vi "FormCalibra7.vi"() -> ()   [LabVIEW 2014]
uses:
  testMachine.ctl
  mainMachine.ctl
  <vilib>/Instr/_visa.llb/VISA Configure Serial Port (Instr).vi
  <vilib>/express/express shared/transition.llb/Dynamic To Waveform Array.vi
  <vilib>/express/express signal manip/GetorSetDDTAttributes/Set DDT Attributes/SetT0.vi
  <vilib>/express/express shared/transition.llb/Waveform Array To Dynamic.vi
  <vilib>/express/express signal manip/GetorSetDDTAttributes/Set DDT Attributes/Set DDT Properties.xnode
panel:
  out "String":string
  in  "VISA Serial Port":refnum<visa-resource-name>
  out "editDistance":dbl caption="Distancia (m)" format="%#_4f"
  in  "Lower level":dbl
  in  "hysteresis":dbl format="%.2p"
  in  "level":dbl format="%.2p"
  out "editTotalWaitLimit":u8
  out "editCountWaitLimit":u8
  out "ledWaitState":bool caption="Wait State"
  out "sliderWaitUpperTime":u8(slide) max=50 scale=0.0..30.0
  out "slideWaitLowerTime":u8(slide) max=30 scale=0.0..1.0
  out "slideWaitTime":u8(slide) scale=0.0..1.0
  out "labelTestTime":string caption="Tempo total de ensaio"
  in  "buttonAcquisition":bool
  in  "editSetWaitTime":u8 caption="Tempo entre ciclos (s)" step=1 format="%0d"
  in  "stop":bool
  out "ledAcquireState":bool caption="Acquire State"
  out "editTotalLowerLimit":u8
  out "editCountLowerLimit":u8
  out "editTotalUpperLimit":u8
  out "editCountUpperLimit":u8
  out "ledEnsaio 3":bool
  out "ledBrakeState":bool caption="Brake State"
  out "ledExitState":bool caption="Exit State"
  out "ledMotorState":bool caption="Motor State"
  out "ledInit2State":bool caption="Init State"
  out "ledBlockState":bool caption="Block State"
  out "ledRunningState":bool caption="Running State"
  out "ledReadyState":bool caption="Ready State"
  out "ledInitState":bool caption="Init State"
  out "mainMachine":T1
  out "testMachine":T2=enum."finish"
  in  "editSetPathToFile":path
  in  "buttonStop":bool
  in  "buttonStart":bool
  out "graphForce":dynamicdata(graph)
  in  "editOffsetForce":dbl caption="Tara" min=0.0 max=100.0 step=0.1
  in  "editSetForce":dbl caption="Fator de conversão"
  out "editForce":dbl caption="Força (Kgf)" format="%#_4f"
  out "graphSpeed":dynamicdata(graph)
  in  "editSetSpeed":dbl caption="Fator de conversão"
  out "editSpeed":dbl caption="Velocidade (km/h)" format="%#_4f"
  out "editEngineSpeed":dbl caption="Rotação (RPM)" format="%#_4f"
  in  "buttonMotor":bool
  in  "buttonBrake":bool
  in  "editSetWaitLowerTime":u8 caption="Tempo de espera (s)"
  in  "editSetWaitUpperTime":u8=3 caption="Tempo de espera (s)"
  in  "editSetNumberOfCycles":u16 caption="Número de ciclos" max=999 step=1 format="%0d"
  in  "editSetLowerLimit":u32 caption="Limite inferior (km/h)"
  in  "editSetUpperLimit":u32 caption="Limite superior (km/h)"
  out "editTempA":dbl caption="Temperatura A (ºC)"
  in  "editSetTempRef":dbl caption="Offset referência" step=0.01 format="%#_2f"
  out "editTempRef":dbl caption="Referência (ºC)"
  out "ledMotor":bool
  out "ledBrake":bool
  out "ledEnsaio":bool
  out "labelTotalCycle":string
  out "labelCurrentCycle":string
  out "labelSystemTitle":string
  in  "editCurrCycleCtr":u32
  in  "velocidade 2":u32
  out "velocidade":u32
  # "Bancada de Frenagem - Ensaio"
  # "Ensaio"
  # "Temperatura"
  # "Rotação"
  # "Célula de Carga"
  # "Configurações do ensaio"
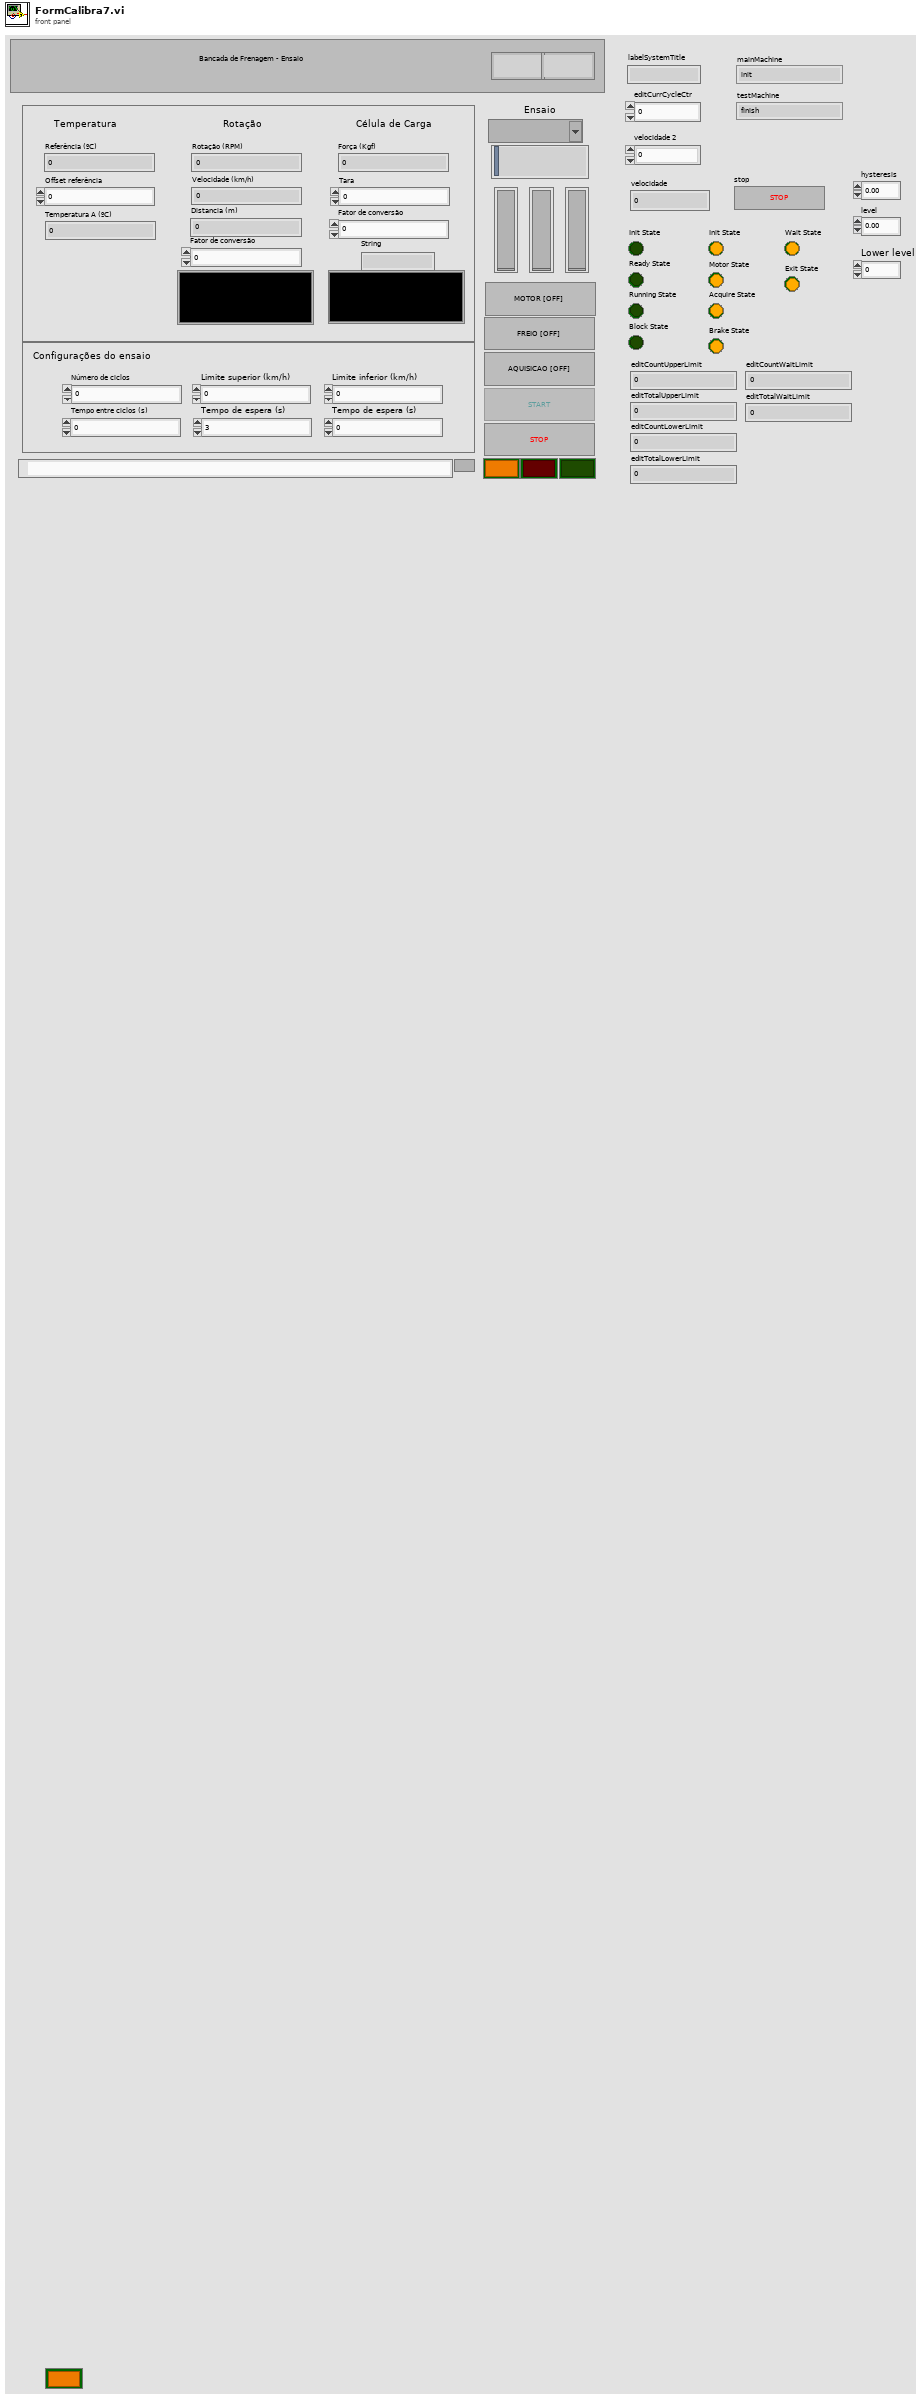
[diagram p1: front panel]
types:
  T1 = typedef "mainMachine.ctl" = enum16{"init", "ready", "running", "blocked", "finish"}
  T2 = typedef "testMachine.ctl" = enum16{"init", "motor", "motor acquire", "brake", "brake acquire", "wait ", "finish", "exit"}
  T3 = enum8{"Enabled", "Disabled", "Disabled and Grayed Out"}
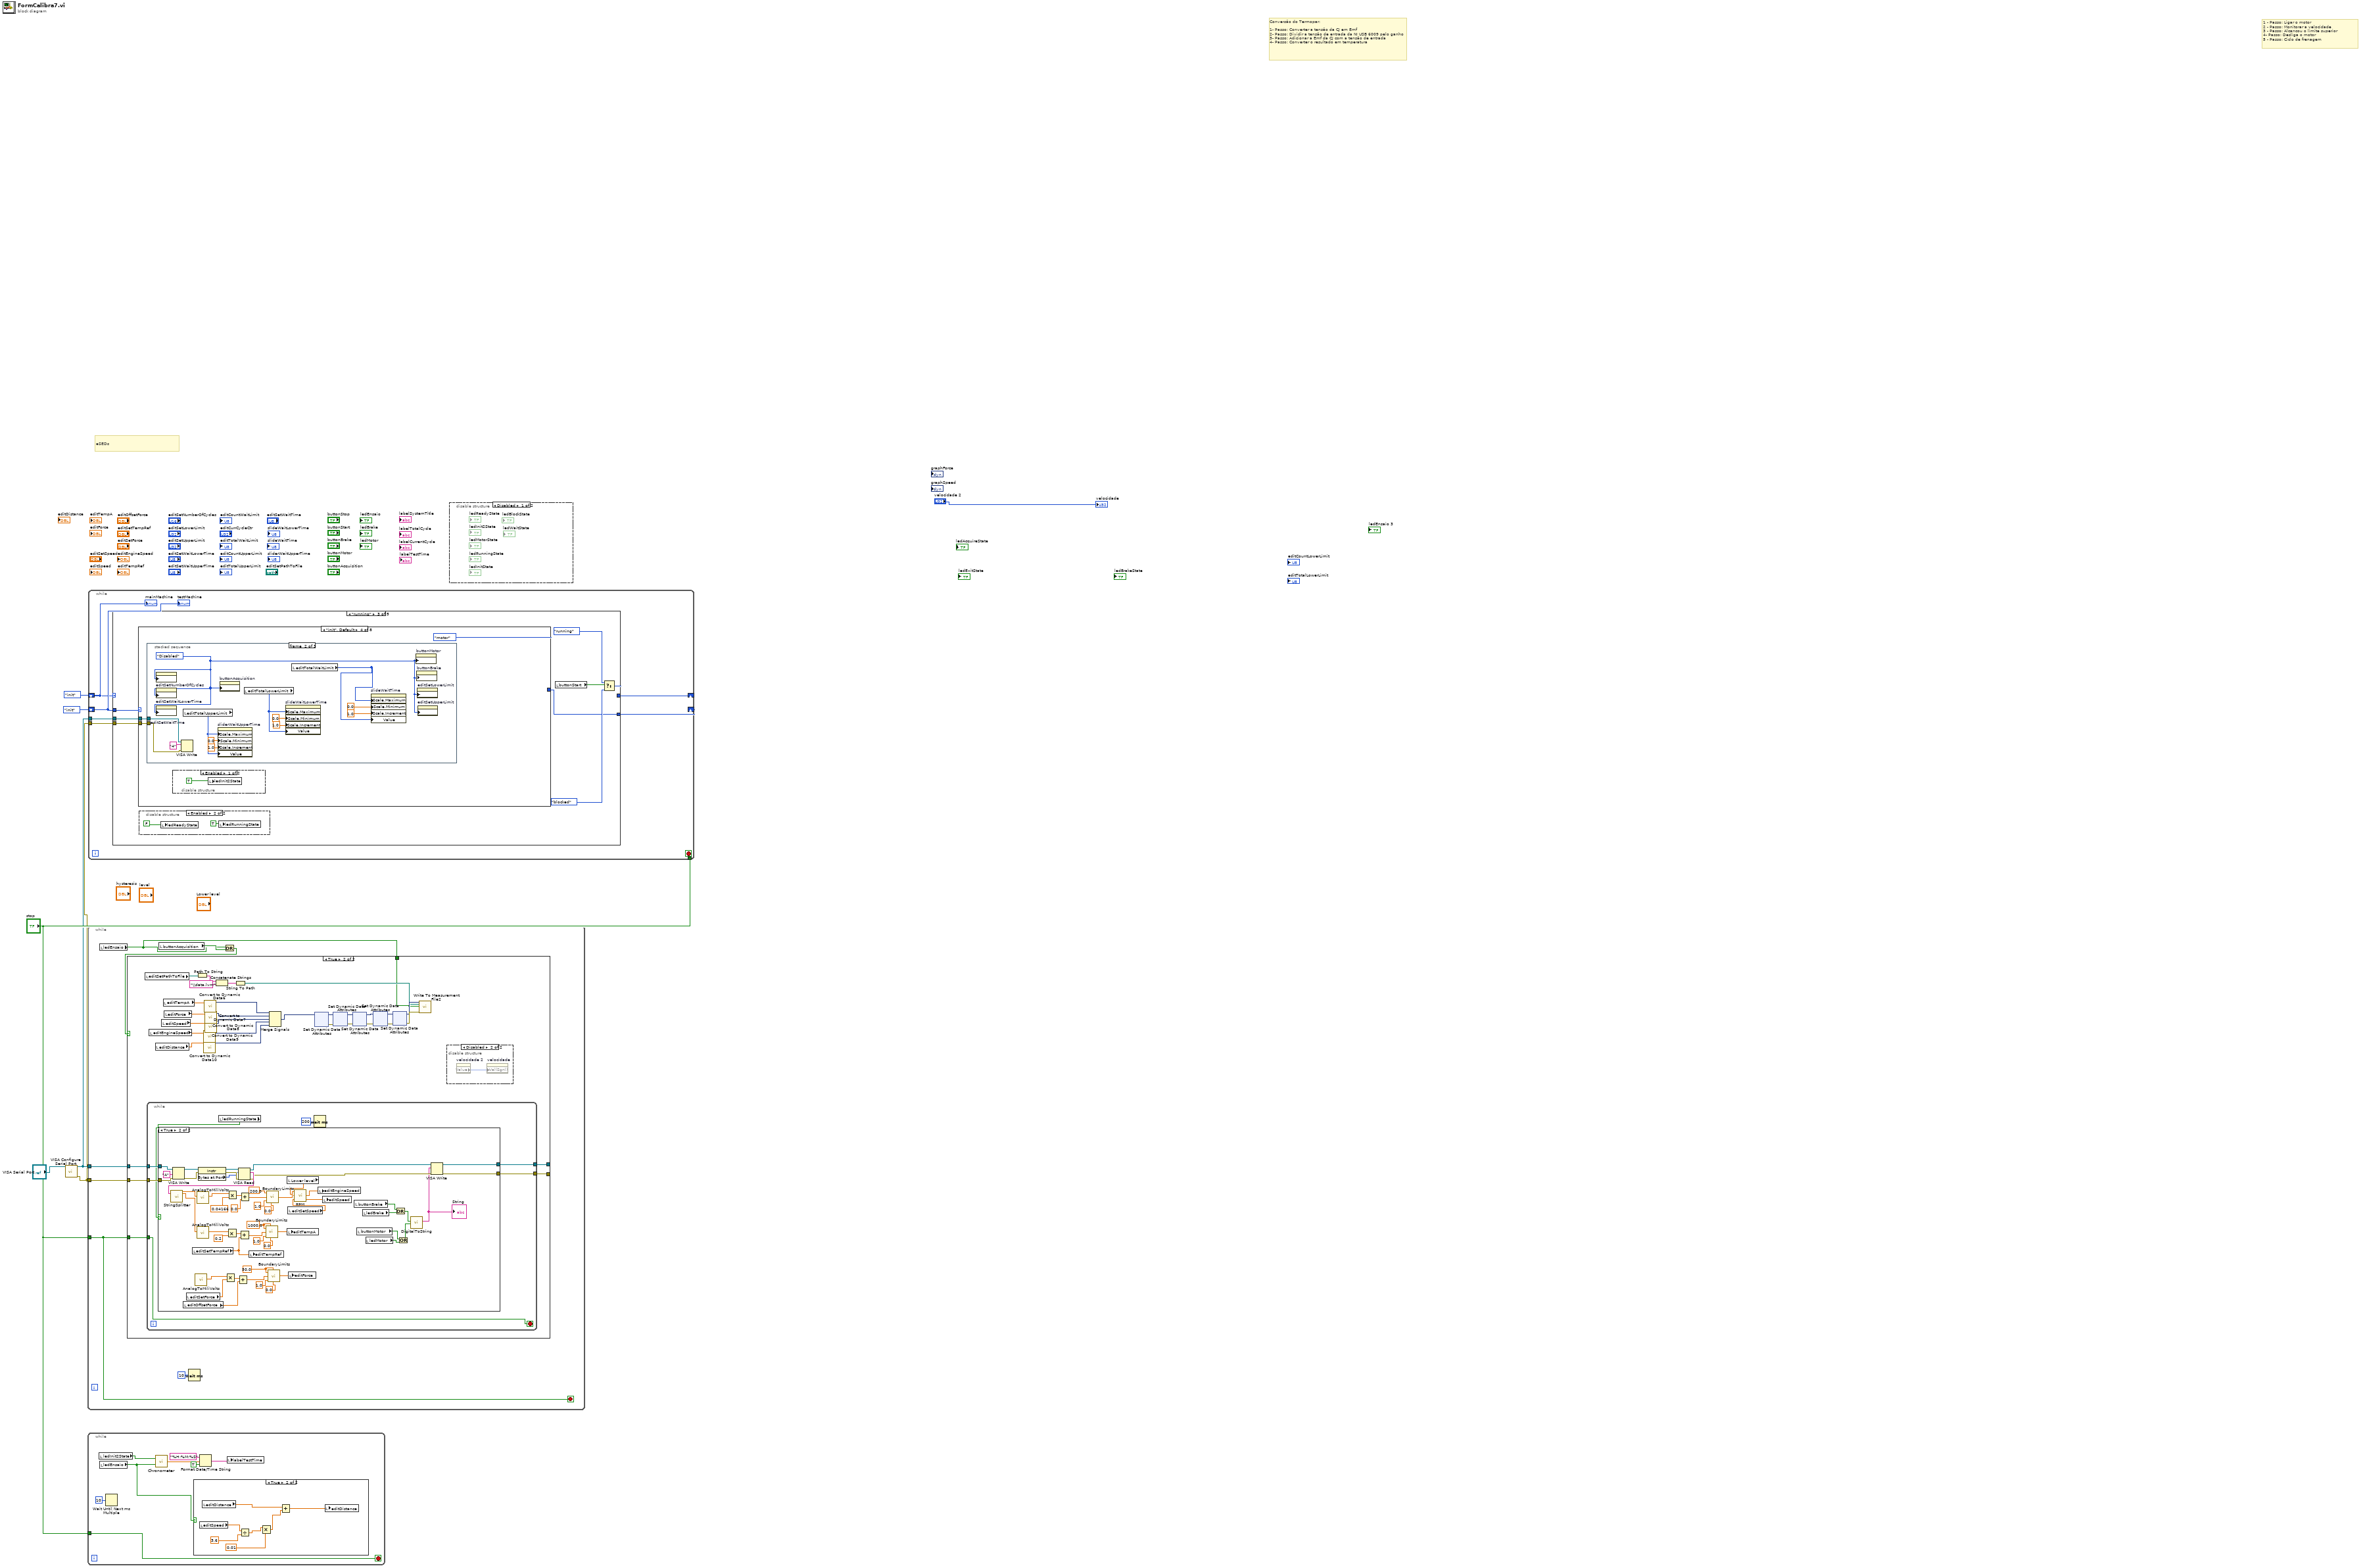
[diagram p0: block diagram]
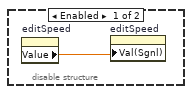
[diagram p6: hidden frame]
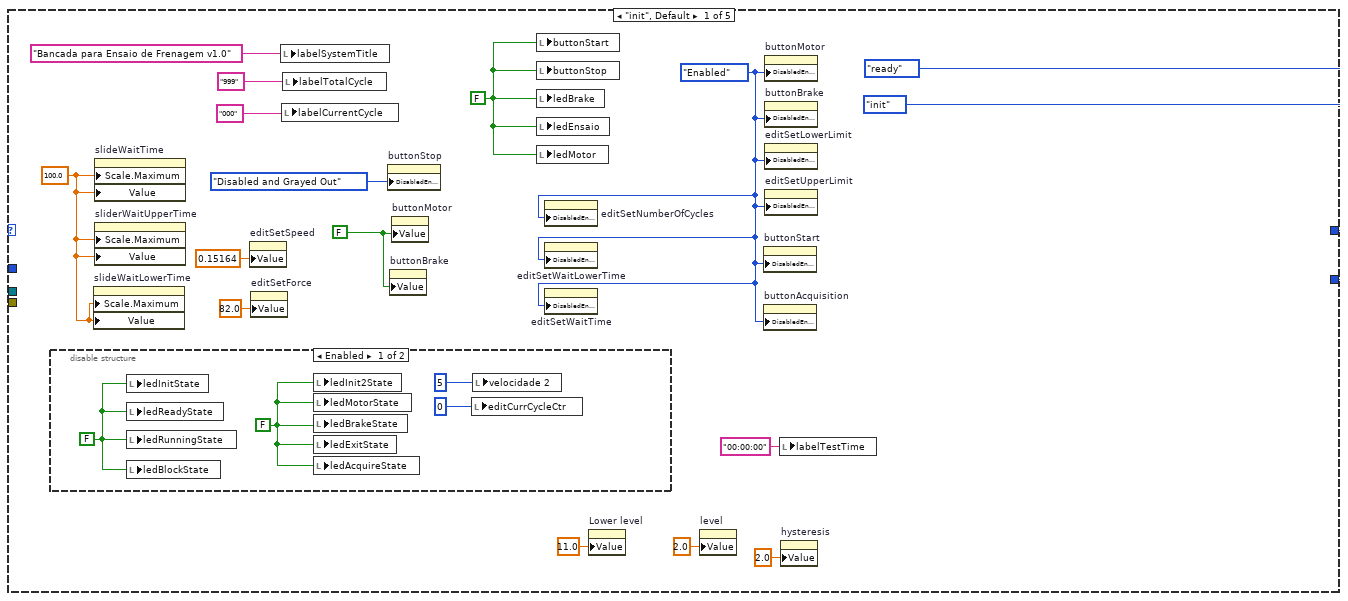
[diagram p7: hidden frame]
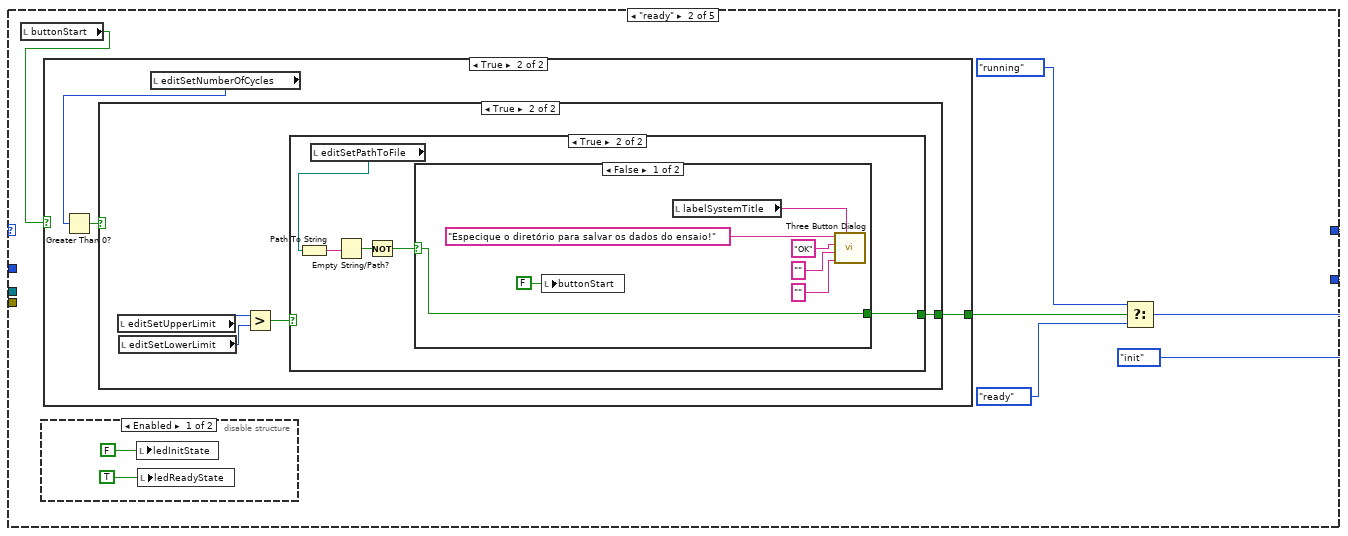
[diagram p9: hidden frame]
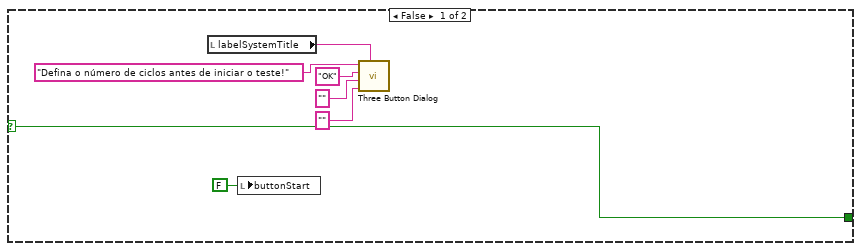
[diagram p12: hidden frame]
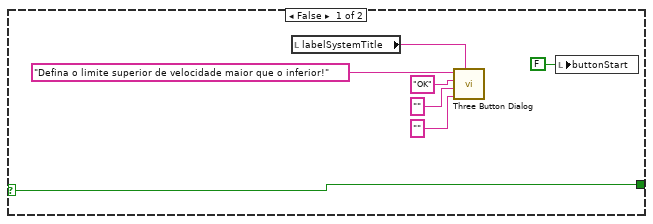
[diagram p13: hidden frame]
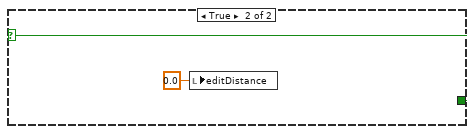
[diagram p14: hidden frame]
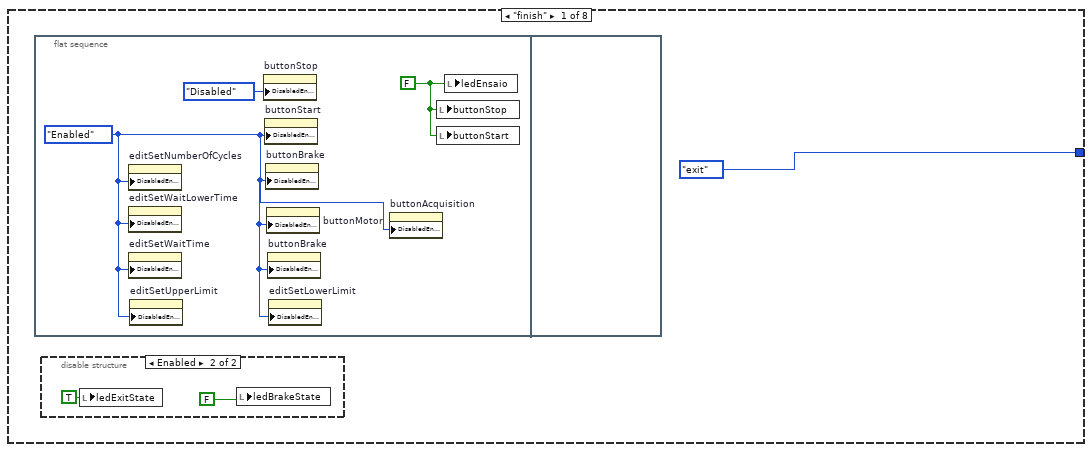
[diagram p16: hidden frame]
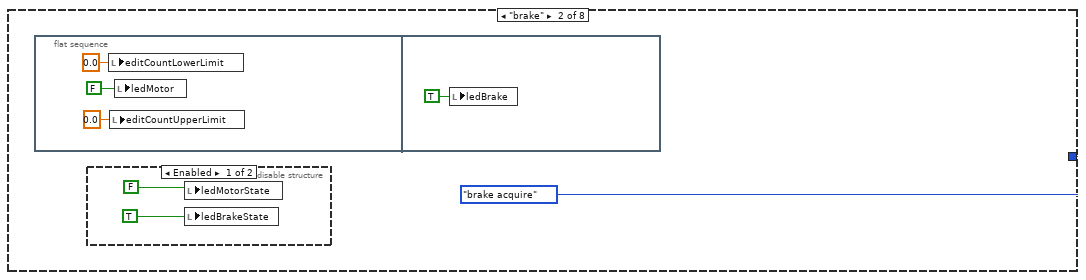
[diagram p18: hidden frame]
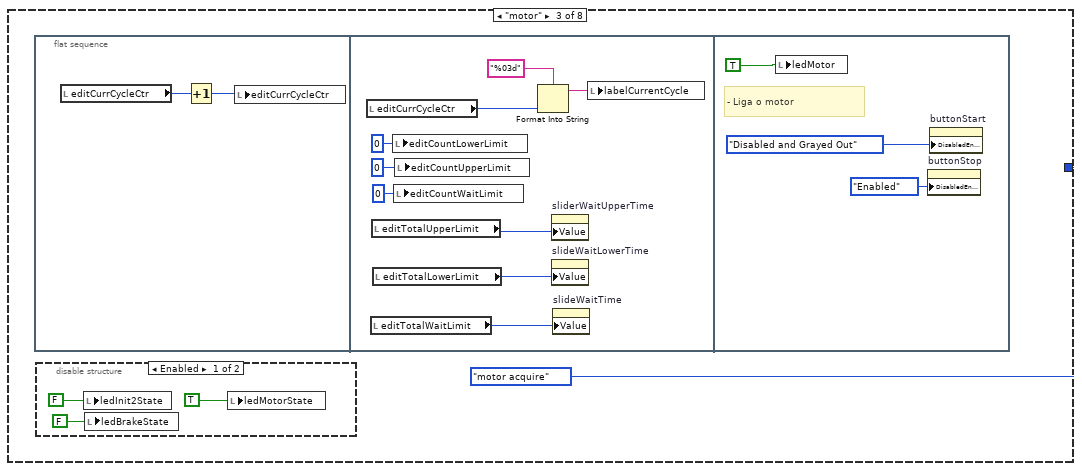
[diagram p20: hidden frame]
diagram:
  # "eSEDs"
  # "1 - Passo: Ligar o motor\n2 - Passo: Monitorar a velocidade\n3 - Passo: Alcancou o limite superior\n4- Passo: Desliga o motor\n5 - Passo: Ciclo de frenagem"
  # "Conversão do Termopar:\n\n1- Passo: Converter a tensão da CJ em Emf\n2- Passo: Dividir a tensão de entrada da NI USB 6009 pelo ganho\n3- Passo: Adicionar a Emf da CJ com a tensão de entrada\n4- Passo: Converter o resultado em temperatura"
  n1 = call-poly "VISA Configure Serial Port"("VISA resource name"="VISA Serial Port") -> ("VISA resource name out"=w2:refnum<visa-resource-name>, "error out"=w1:errorcluster)  [unwired: 13 in]
  n2 = while {
    tunnel: "stop" -> [w15]
    stop <- w15 stop-if-true
    n3 = local read "ledInit2State"() -> (w10:bool)
    n4 = local read "ledEnsaio"() -> (w8:bool)
    n5 = Wait Until Next ms Multiple(millisecond multiple=u32 10) -> ()  [unwired: 1 out]
    n6 = call "Chronometer.vi"("start"=w8, "reset"=w10) -> ("Time"=w14:dbl)
    n7 = case shown="True" w8 {
      frame False {
      }
      frame True {
        n8 = local read "editSpeed"() -> (w20:dbl)
        n9 = local read "editDistance"() -> (w22:dbl)
        n10 = Divide(x=w20, y=3.6) -> (x/y=w18:dbl)
        n11 = Multiply(x=w18, y=0.01) -> (x*y=w17:dbl)
        n12 = Add(x=w22, y=w17) -> (x+y=w16:dbl)
        n13 = local write "editDistance"(w16) -> ()
      }
    }
    n14 = Format Date/Time String(time format string (%c)="%H:%M:%S", seconds (now)=w14, UTC format=TRUE) -> (date/time string=w11:string)
    n15 = local write "labelTestTime"(w11) -> ()
  }
  n16 = while {
    tunnel: "stop" -> [w23]
    tunnel: w2 -> [w25]
    tunnel: w1 -> [w24]
    stop <- w23 stop-if-true
    n17 = local read "ledEnsaio"() -> (w27:bool)
    n18 = local read "buttonAcquisition"() -> (w29:bool)
    n19 = Wait (ms)(milliseconds to wait=u32 10) -> ()  [unwired: 1 out]
    n20 = Or(x=w27, y=w29) -> (x .or. y?=w28:bool)
    n21 = case shown="True" w28 {
      tunnel: w27 -> [_ w41]
      tunnel: w25 -> [w31 w36]
      tunnel: w24 -> [w30 w35]
      tunnel: [w31 w34] -> _
      tunnel: [w30 w33] -> _
      tunnel: w23 -> [_ w32]
      frame False {
      }
      frame True {
        n22 = local read "editSetPathToFile"() -> (w43:path)
        n23 = while {
          tunnel: w36 -> [w69]
          tunnel: w35 -> [w68]
          tunnel: [w67] -> w34
          tunnel: [w66] -> w33
          tunnel: w32 -> [w65]
          stop <- w65 stop-if-true
          n24 = local read "ledRunningState"() -> (w64:bool)
          n25 = case shown="True" w64 {
            tunnel: w69 -> [w72 w78]
            tunnel: w68 -> [w71 w77]
            tunnel: [w72 w75] -> w67
            tunnel: [w71 w74] -> w66
            frame False {
            }
            frame True {
              w98 = 50.0
              w108 = 1000.0
              n26 = VISA Write(VISA resource name=w78, write buffer="A", error in (no error)=w77) -> (VISA resource name out=w125:refnum<visa-resource-name>, error out=w124:errorcluster)  [unwired: 1 out]
              n27 = local read "editOffsetForce"() -> (w93:dbl)
              n28 = local read "editSetForce"() -> (w94:dbl)
              n29 = local read "editSetTempRef"() -> (w101:dbl)
              n30 = call "AnalogToMiliVolts.vi"() -> ("Output"=w99:dbl)  [unwired: 11 in]
              n31 = property class="Instr"(reference=w125, error in=w124) -> (reference out=w123:refnum<visa-resource-name>, error out=w122:errorcluster, "Bytes at Port"=w121:u32)
              n32 = Multiply(x=w99, y=w94) -> (x*y=w100:dbl)
              n33 = Add(x=w100, y=w93) -> (x+y=w95:dbl)
              n34 = VISA Read(VISA resource name=w123, byte count=w121, error in (no error)=w122) -> (VISA resource name out=w85:refnum<visa-resource-name>, read buffer=w102:string, error out=w86:errorcluster)  [unwired: 1 out]
              n35 = call "StringSplitter.vi"("Input String"=w102) -> ("S0"=w104:dbl, "S1"=w103:dbl)  [unwired: 11 in, 6 out]
              n36 = call "AnalogToMiliVolts.vi"("Input"=w104) -> ("Output"=w117:dbl)  [unwired: 10 in]
              n37 = call "AnalogToMiliVolts.vi"("Input"=w103) -> ("Output"=w109:dbl)  [unwired: 10 in]
              n38 = Multiply(x=w109, y=0.2) -> (x*y=w110:dbl)
              n39 = Multiply(x=w117, y=0.04166) -> (x*y=w118:dbl)
              n40 = Add(x=w110, y=w101) -> (x+y=w105:dbl)
              n41 = Add(x=w118, y=0.0) -> (x+y=w116:dbl)
              n42 = local write "editTempRef"(w101) -> ()
              n43 = call "BoundaryLimits.vi"("UpperLimit"=w108, "UpperValue"=w108, "Input"=w105, "LowerLimit"=1.0, "LowerValue"=0.0) -> ("Output"=w92:dbl)
              n44 = call "BoundaryLimits.vi"("UpperLimit"=200.0, "Input"=w116, "LowerLimit"=1.0, "LowerValue"=0.0) -> ("Output"=w91:dbl)  [unwired: 1 in]
              n45 = call "BoundaryLimits.vi"("UpperLimit"=w98, "UpperValue"=w98, "Input"=w95, "LowerLimit"=1.0, "LowerValue"=0.0) -> ("Output"=w76:dbl)
              n46 = local read "Lower level"() -> (w90:dbl)
              n47 = local write "editTempA"(w92) -> ()
              n48 = local read "editSetSpeed"() -> (w89:dbl)
              n49 = local write "editForce"(w76) -> ()
              n50 = call "RPM.vi"("factor"=w89, "Lower level"=w90, "data"=w91) -> ("km/h"=w88:dbl, "RPM"=w87:dbl)  [unwired: 1 out]
              n51 = local write "editEngineSpeed"(w87) -> ()
              n52 = local write "editSpeed"(w88) -> ()
              n53 = local read "buttonBrake"() -> (w82:bool)
              n54 = local read "buttonMotor"() -> (w84:bool)
              n55 = local read "ledBrake"() -> (w81:bool)
              n56 = local read "ledMotor"() -> (w83:bool)
              n57 = Or(x=w82, y=w81) -> (x .or. y?=w80:bool)
              n58 = Or(x=w84, y=w83) -> (x .or. y?=w79:bool)
              n59 = call "DigitalToString.vi"("D1"=w79, "D0"=w80) -> ("Out"=w73:string)  [unwired: 9 in]
              "String" <- w73
              n60 = VISA Write(VISA resource name=w85, write buffer=w73, error in (no error)=w86) -> (VISA resource name out=w75:refnum<visa-resource-name>, error out=w74:errorcluster)  [unwired: 1 out]
            }
          }
          n61 = Wait (ms)(milliseconds to wait=u32 200) -> ()  [unwired: 1 out]
        }
        n62 = local read "editEngineSpeed"() -> (w39:dbl)
        n63 = local read "editDistance"() -> (w40:dbl)
        n64 = local read "editSpeed"() -> (w37:dbl)
        n65 = local read "editTempA"() -> (w55:dbl)
        n66 = local read "editForce"() -> (w38:dbl)
        n67 = Path To String(path=w43) -> (string=w42:string)
        n68 = call "Convert to Dynamic Data9"("Double"=w39) -> ("Dynamic Data Type"=w59:dynamicdata)  [unwired: 3 in]
        n69 = call "Convert to Dynamic Data10"("Double"=w40) -> ("Dynamic Data Type"=w60:dynamicdata)  [unwired: 3 in]
        n70 = call "Convert to Dynamic Data6"("Double"=w55) -> ("Dynamic Data Type"=w56:dynamicdata)  [unwired: 3 in]
        n71 = call "Convert to Dynamic Data7"("Double"=w38) -> ("Dynamic Data Type"=w57:dynamicdata)  [unwired: 3 in]
        n72 = call "Convert to Dynamic Data8"("Double"=w37) -> ("Dynamic Data Type"=w58:dynamicdata)  [unwired: 3 in]
        n73 = Concatenate Strings(w42, "\\data.lvm" ("string")) -> (w45:string)
        n74 = String To Path(string=w45) -> (path=w46:path)
        n75 = Merge Signals(w56, w57, w58, w59, w60) -> (w61:dynamicdata)
        n76 = xnode ("Set Dynamic Data Attributes")("Signals In"=w61) -> ("Signals Out"=w47:dynamicdata, "error out"=w49:errorcluster)  [unwired: 4 in]
        n77 = xnode ("Set Dynamic Data Attributes")("Signals In"=w47, "error in"=w49) -> ("Signals Out"=w48:dynamicdata, "error out"=w50:errorcluster)  [unwired: 3 in]
        n78 = xnode ("Set Dynamic Data Attributes")("Signals In"=w48, "error in"=w50) -> ("Signals Out"=w62:dynamicdata, "error out"=w51:errorcluster)  [unwired: 3 in]
        n79 = xnode ("Set Dynamic Data Attributes")("Signals In"=w62, "error in"=w51) -> ("Signals Out"=w63:dynamicdata, "error out"=w52:errorcluster)  [unwired: 3 in]
        n80 = xnode ("Set Dynamic Data Attributes")("Signals In"=w63, "error in"=w52) -> ("Signals Out"=w53:dynamicdata, "error out"=w54:errorcluster)  [unwired: 3 in]
        n81 = call "Write To Measurement File2"("Signals"=w53, "Enable"=w41, "error in (no error)"=w54, "Filename"=w46) -> ()  [unwired: 13 in, 3 out]
        n82 = disable-structure shown="Disabled" {
          frame Enabled {
            n83 = property on="editSpeed" class="DigNum (strict)"() -> ("Value"=w126:dbl)  [unwired: 2 in, 2 out]
            n84 = property on="editSpeed" class="DigNum (strict)"("Val(Sgnl)"=w126) -> ()  [unwired: 2 in, 2 out]
          }
          frame Disabled {
            n85 = property on="velocidade 2" class="DigNum (strict)"() -> ("Value"=w127:u32)  [unwired: 2 in, 2 out]
            n86 = property on="velocidade" class="DigNum (strict)"("Val(Sgnl)"=w127) -> ()  [unwired: 2 in, 2 out]
          }
        }
      }
    }
  }
  n87 = while {
    shift-right: [w224] -> _
    shift-left: mainMachine."init" ("mainMachine") -> [w221]
    shift-right: [w223] -> _
    shift-left: testMachine."init" ("testMachine") -> [w222]
    tunnel: "stop" -> [w220]
    tunnel: w2 -> [w219]
    tunnel: w1 -> [w218]
    stop <- w220 stop-if-true
    n88 = case shown="\"running\"" w221 {
      tunnel: [mainMachine."ready" ("mainMachine") w245 w293 w435 mainMachine."finish" ("mainMachine")] -> w224
      tunnel: [testMachine."init" ("testMachine") testMachine."init" ("testMachine") w292 testMachine."init" ("testMachine") testMachine."init" ("testMachine")] -> w223
      tunnel: w222 -> [_ _ w291 _ _]
      tunnel: w219 -> [_ _ w290 _ _]
      tunnel: w218 -> [_ _ w289 _ _]
      frame "init", Default {
        w231 = 100.0 ("Scale.Range:Maximum")
        w232 = T3."Enabled" ("Disabled")
        w233 = FALSE ("buttonMotor")
        w239 = FALSE ("motor")
        n89 = disable-structure shown="Enabled" {
          frame Enabled {
            w241 = FALSE
            w242 = FALSE
            n90 = local write "ledInitState"(w242) -> ()
            n91 = local write "ledReadyState"(w242) -> ()
            n92 = local write "ledRunningState"(w242) -> ()
            n93 = local write "ledBlockState"(w242) -> ()
            n94 = local write "ledInit2State"(w241) -> ()
            n95 = local write "ledMotorState"(w241) -> ()
            n96 = local write "ledBrakeState"(w241) -> ()
            n97 = local write "ledExitState"(w241) -> ()
            n98 = local write "ledAcquireState"(w241) -> ()
            n99 = local write "editCurrCycleCtr"(u32 0 ("currentCycleCtr")) -> ()
            n100 = local write "velocidade 2"(u32 5 ("velocidade 2")) -> ()
          }
          frame Disabled {
          }
        }
        n101 = property on="slideWaitLowerTime" class="Slide (strict)"("Scale.Maximum"=w231, "Value"=w231) -> ()  [unwired: 2 in, 2 out]
        n102 = property on="slideWaitTime" class="Slide (strict)"("Scale.Maximum"=w231, "Value"=w231) -> ()  [unwired: 2 in, 2 out]
        n103 = property on="sliderWaitUpperTime" class="Slide (strict)"("Scale.Maximum"=w231, "Value"=w231) -> ()  [unwired: 2 in, 2 out]
        n104 = property on="editSetSpeed" class="DigNum (strict)"("Value"=0.15164 ("editSetSpeed")) -> ()  [unwired: 2 in, 2 out]
        n105 = property on="editSetForce" class="DigNum (strict)"("Value"=82.0 ("editSetForce")) -> ()  [unwired: 2 in, 2 out]
        n106 = local write "labelSystemTitle"("Bancada para Ensaio de Frenagem v1.0" ("systemTitle")) -> ()
        n107 = local write "labelCurrentCycle"("000" ("currentCycle")) -> ()
        n108 = local write "labelTotalCycle"("999" ("totalCycle")) -> ()
        n109 = property on="buttonStop" class="Bool (strict)"("DisabledEnum"=T3."Disabled and Grayed Out" ("Disabled")) -> ()  [unwired: 2 in, 2 out]
        n110 = property on="buttonBrake" class="Bool (strict)"("Value"=w233) -> ()  [unwired: 2 in, 2 out]
        n111 = property on="buttonMotor" class="Bool (strict)"("Value"=w233) -> ()  [unwired: 2 in, 2 out]
        n112 = local write "buttonStart"(w239) -> ()
        n113 = local write "buttonStop"(w239) -> ()
        n114 = local write "ledBrake"(w239) -> ()
        n115 = local write "ledEnsaio"(w239) -> ()
        n116 = local write "ledMotor"(w239) -> ()
        n117 = property on="editSetNumberOfCycles" class="DigNum (strict)"("DisabledEnum"=w232) -> ()  [unwired: 2 in, 2 out]
        n118 = property on="editSetWaitLowerTime" class="DigNum (strict)"("DisabledEnum"=w232) -> ()  [unwired: 2 in, 2 out]
        n119 = property on="editSetWaitTime" class="DigNum (strict)"("DisabledEnum"=w232) -> ()  [unwired: 2 in, 2 out]
        n120 = property on="Lower level" class="DigNum (strict)"("Value"=11.0 ("Lower level")) -> ()  [unwired: 2 in, 2 out]
        n121 = property on="level" class="DigNum (strict)"("Value"=2.0 ("level")) -> ()  [unwired: 2 in, 2 out]
        n122 = property on="buttonStart" class="Bool (strict)"("DisabledEnum"=w232) -> ()  [unwired: 2 in, 2 out]
        n123 = property on="buttonAcquisition" class="Bool (strict)"("DisabledEnum"=w232) -> ()  [unwired: 2 in, 2 out]
        n124 = property on="buttonMotor" class="Bool (strict)"("DisabledEnum"=w232) -> ()  [unwired: 2 in, 2 out]
        n125 = property on="buttonBrake" class="Bool (strict)"("DisabledEnum"=w232) -> ()  [unwired: 2 in, 2 out]
        n126 = property on="editSetLowerLimit" class="DigNum (strict)"("DisabledEnum"=w232) -> ()  [unwired: 2 in, 2 out]
        n127 = property on="editSetUpperLimit" class="DigNum (strict)"("DisabledEnum"=w232) -> ()  [unwired: 2 in, 2 out]
        n128 = local write "labelTestTime"("00:00:00" ("labelTestTime")) -> ()
        n129 = property on="hysteresis" class="DigNum (strict)"("Value"=2.0 ("hysteresis")) -> ()  [unwired: 2 in, 2 out]
      }
      frame "ready" {
        n130 = local read "buttonStart"() -> (w248:bool)
        n131 = disable-structure shown="Enabled" {
          frame Enabled {
            n132 = local write "ledInitState"(FALSE ("ledReady")) -> ()
            n133 = local write "ledReadyState"(TRUE ("ledReady")) -> ()
          }
          frame Disabled {
          }
        }
        n134 = case shown="True" w248 {
          selector: w248 -> [w253 _]
          tunnel: [w253 w254] -> w247
          frame False {
          }
          frame True {
            n135 = local read "editSetNumberOfCycles"() -> (w255:u16)
            n136 = Greater Than 0?(x=w255) -> (x > 0?=w256:bool)
            n137 = case shown="True" w256 {
              selector: w256 -> [w263 _]
              tunnel: [w263 w264] -> w254
              frame False {
                n138 = local read "labelSystemTitle"() -> (w258:string)
                n139 = local write "buttonStart"(FALSE ("startButton")) -> ()
                n140 = call <vilib>:"Three Button Dialog.vi"("Window Title (\"\")"=w258, "Right Button Text (\"Cancel\")"="" ("Right Button Text (\"Cancel\")"), "Center Button Text (\"No\")"="" ("Center Button Text (\"No\")"), "Left Button Text (\"Yes\")"="OK" ("Left Button Text (\"Yes\")"), "message"="Defina o número de ciclos antes de iniciar o teste!") -> ()  [unwired: 6 in, 1 out]
              }
              frame True {
                n141 = local read "editSetUpperLimit"() -> (w266:u32)
                n142 = local read "editSetLowerLimit"() -> (w265:u32)
                n143 = Greater?(x=w266, y=w265) -> (0:w267:bool)
                n144 = case shown="True" w267 {
                  selector: w267 -> [w274 _]
                  tunnel: [w274 w277] -> w264
                  frame False {
                    n145 = local read "labelSystemTitle"() -> (w269:string)
                    n146 = call <vilib>:"Three Button Dialog.vi"("Window Title (\"\")"=w269, "Right Button Text (\"Cancel\")"="" ("Right Button Text (\"Cancel\")"), "Center Button Text (\"No\")"="" ("Center Button Text (\"No\")"), "Left Button Text (\"Yes\")"="OK" ("Left Button Text (\"Yes\")"), "message"="Defina o limite superior de velocidade maior que o inferior!") -> ()  [unwired: 6 in, 1 out]
                    n147 = local write "buttonStart"(FALSE ("startButton")) -> ()
                  }
                  frame True {
                    n148 = local read "editSetPathToFile"() -> (w279:path)
                    n149 = Path To String(path=w279) -> (string=w278:string)
                    n150 = Empty String/Path?(string/path=w278) -> (empty?=w276:bool)
                    n151 = Not(x=w276) -> (.not. x?=w275:bool)
                    n152 = case shown="False" w275 {
                      selector: w275 -> [w286 w288]
                      tunnel: [w286 w288] -> w277
                      frame False {
                        n153 = local write "buttonStart"(FALSE ("startButton")) -> ()
                        n154 = local read "labelSystemTitle"() -> (w281:string)
                        n155 = call <vilib>:"Three Button Dialog.vi"("Window Title (\"\")"=w281, "Right Button Text (\"Cancel\")"="" ("Right Button Text (\"Cancel\")"), "Center Button Text (\"No\")"="" ("Center Button Text (\"No\")"), "Left Button Text (\"Yes\")"="OK" ("Left Button Text (\"Yes\")"), "message"="Especique o diretório para salvar os dados do ensaio!") -> ()  [unwired: 6 in, 1 out]
                      }
                      frame True {
                        n156 = local write "editDistance"(0.0 ("editDistance")) -> ()
                      }
                    }
                  }
                }
              }
            }
          }
        }
        n157 = Select(t=mainMachine."running" ("mainMachine"), s=w247, f=mainMachine."ready" ("mainMachine")) -> (s? t:f=w245:T1)
      }
      frame "running" {
        n158 = case shown="\"init\", Default" w291 {
          tunnel: [testMachine."exit" ("testMachine") testMachine."brake acquire" ("testMachine") testMachine."motor acquire" ("testMachine") testMachine."motor" ("testMachine") w365 w385 testMachine."exit" ("testMachine") w418] -> w292
          tunnel: w290 -> [_ _ _ w331 _ _ _ _]
          tunnel: w289 -> [_ _ _ w330 _ _ _ _]
          frame "finish" {
            n159 = flat-sequence {
              frame #0 {
                w303 = FALSE ("ledReady")
                w302 = T3."Enabled" ("Disabled")
                n160 = property on="editSetNumberOfCycles" class="DigNum (strict)"("DisabledEnum"=w302) -> ()  [unwired: 2 in, 2 out]
                n161 = property on="editSetWaitLowerTime" class="DigNum (strict)"("DisabledEnum"=w302) -> ()  [unwired: 2 in, 2 out]
                n162 = property on="editSetWaitTime" class="DigNum (strict)"("DisabledEnum"=w302) -> ()  [unwired: 2 in, 2 out]
                n163 = property on="editSetUpperLimit" class="DigNum (strict)"("DisabledEnum"=w302) -> ()  [unwired: 2 in, 2 out]
                n164 = property on="buttonStop" class="Bool (strict)"("DisabledEnum"=T3."Disabled" ("Disabled")) -> ()  [unwired: 2 in, 2 out]
                n165 = property on="buttonStart" class="Bool (strict)"("DisabledEnum"=w302) -> ()  [unwired: 2 in, 2 out]
                n166 = property on="buttonBrake" class="Bool (strict)"("DisabledEnum"=w302) -> ()  [unwired: 2 in, 2 out]
                n167 = property on="buttonMotor" class="Bool (strict)"("DisabledEnum"=w302) -> ()  [unwired: 2 in, 2 out]
                n168 = property on="buttonBrake" class="Bool (strict)"("DisabledEnum"=w302) -> ()  [unwired: 2 in, 2 out]
                n169 = property on="editSetLowerLimit" class="DigNum (strict)"("DisabledEnum"=w302) -> ()  [unwired: 2 in, 2 out]
                n170 = property on="buttonAcquisition" class="Bool (strict)"("DisabledEnum"=w302) -> ()  [unwired: 2 in, 2 out]
                n171 = local write "buttonStop"(w303) -> ()
                n172 = local write "buttonStart"(w303) -> ()
                n173 = local write "ledEnsaio"(w303) -> ()
              }
              frame #1 {
              }
            }
            n174 = disable-structure shown="Enabled" {
              frame Disabled {
              }
              frame Enabled {
                n175 = local write "ledExitState"(TRUE ("ledReady")) -> ()
                n176 = local write "ledBrakeState"(FALSE ("ledReady")) -> ()
              }
            }
          }
          frame "brake" {
            n177 = flat-sequence {
              frame #0 {
                n178 = local write "editCountLowerLimit"(0.0 ("editCountUpperLimit")) -> ()
                n179 = local write "editCountUpperLimit"(0.0 ("editCountUpperLimit")) -> ()
                n180 = local write "ledMotor"(FALSE ("motor")) -> ()
              }
              frame #1 {
                n181 = local write "ledBrake"(TRUE ("freio")) -> ()
              }
            }
            n182 = disable-structure shown="Enabled" {
              frame Enabled {
                n183 = local write "ledMotorState"(FALSE ("ledReady")) -> ()
                n184 = local write "ledBrakeState"(TRUE ("ledReady")) -> ()
              }
              frame Disabled {
              }
            }
          }
          frame "motor" {
            n185 = flat-sequence {
              frame #0 {
                n186 = local read "editCurrCycleCtr"() -> (w317:u32)
                n187 = Increment(x=w317) -> (x+1=w316:u32)
                n188 = local write "editCurrCycleCtr"(w316) -> ()
              }
              frame #1 {
                n189 = local read "editCurrCycleCtr"() -> (w324:u32)
                n190 = local read "editTotalWaitLimit"() -> (w318:u8)
                n191 = local read "editTotalUpperLimit"() -> (w320:u8)
                n192 = local read "editTotalLowerLimit"() -> (w319:u8)
                n193 = local write "editCountLowerLimit"(u8 0 ("editCountLowerLimit")) -> ()
                n194 = local write "editCountWaitLimit"(u8 0 ("editCountWaitLimit")) -> ()
                n195 = local write "editCountUpperLimit"(u8 0 ("editCountUpperLimit")) -> ()
                n196 = Format Into String(format string="%03d", w324) -> (resulting string=w325:string)  [unwired: 2 in, 1 out]
                n197 = property on="sliderWaitUpperTime" class="Slide (strict)"("Value"=w320) -> ()  [unwired: 2 in, 2 out]
                n198 = property on="slideWaitLowerTime" class="Slide (strict)"("Value"=w319) -> ()  [unwired: 2 in, 2 out]
                n199 = property on="slideWaitTime" class="Slide (strict)"("Value"=w318) -> ()  [unwired: 2 in, 2 out]
                n200 = local write "labelCurrentCycle"(w325) -> ()
              }
              frame #2 {
                # "- Liga o motor"
                n201 = local write "ledMotor"(TRUE ("motor")) -> ()
                n202 = property on="buttonStop" class="Bool (strict)"("DisabledEnum"=T3."Enabled" ("Disabled")) -> ()  [unwired: 2 in, 2 out]
                n203 = property on="buttonStart" class="Bool (strict)"("DisabledEnum"=T3."Disabled and Grayed Out" ("Disabled")) -> ()  [unwired: 2 in, 2 out]
              }
            }
            n204 = disable-structure shown="Enabled" {
              frame Enabled {
                n205 = local write "ledInit2State"(FALSE ("ledReady")) -> ()
                n206 = local write "ledBrakeState"(FALSE ("ledReady")) -> ()
                n207 = local write "ledMotorState"(TRUE ("ledReady")) -> ()
              }
              frame Disabled {
              }
            }
          }
          frame "init", Default {
            n208 = stacked-sequence {
              tunnel: w331 -> [_ w350 _]
              tunnel: w330 -> [_ w349 _]
              frame #0 {
                w339 = FALSE ("ensaio")
                n209 = property on="buttonBrake" class="Bool (strict)"("Value"=w339) -> ()  [unwired: 2 in, 2 out]
                n210 = local write "ledMotor"(w339) -> ()
                n211 = local write "ledBrake"(w339) -> ()
                n212 = property on="buttonMotor" class="Bool (strict)"("Value"=w339) -> ()  [unwired: 2 in, 2 out]
                n213 = local read "editSetNumberOfCycles"() -> (w346:u16)
                n214 = local read "editSetWaitLowerTime"() -> (w340:u8)
                n215 = local read "editSetWaitUpperTime"() -> (w343:u8)
                n216 = local read "editSetWaitTime"() -> (w334:u8)
                n217 = Multiply(x=w334, y=u32 10) -> (x*y=w335:u32)
                n218 = Multiply(x=w340, y=u32 10) -> (x*y=w338:u32)
                n219 = Format Into String(format string="%03d", w346) -> (resulting string=w347:string)  [unwired: 2 in, 1 out]
                n220 = Multiply(x=w343, y=u32 10) -> (x*y=w337:u32)
                n221 = local write "editTotalLowerLimit"(w338) -> ()
                n222 = local write "editTotalUpperLimit"(w337) -> ()
                n223 = local write "editTotalWaitLimit"(w335) -> ()
                n224 = local write "labelTotalCycle"(w347) -> ()
                n225 = local write "editCurrCycleCtr"(u32 0 ("currentCycleCtr")) -> ()
                n226 = local write "labelCurrentCycle"("000" ("currentCycle")) -> ()
              }
              frame #1 {
                w358 = T3."Disabled" ("Disabled")
                n227 = property on="editSetNumberOfCycles" class="DigNum (strict)"("DisabledEnum"=w358) -> ()  [unwired: 2 in, 2 out]
                n228 = property on="editSetWaitLowerTime" class="DigNum (strict)"("DisabledEnum"=w358) -> ()  [unwired: 2 in, 2 out]
                n229 = property on="editSetWaitTime" class="DigNum (strict)"("DisabledEnum"=w358) -> ()  [unwired: 2 in, 2 out]
                n230 = VISA Write(VISA resource name=w350, write buffer="4", error in (no error)=w349) -> ()  [unwired: 3 out]
                n231 = local read "editTotalUpperLimit"() -> (w361:u8)
                n232 = property on="sliderWaitUpperTime" class="Slide (strict)"("Scale.Maximum"=w361, "Scale.Minimum"=0.0 ("Scale.Range:Minimum"), "Scale.Increment"=1.0 ("Scale.Range:Increment"), "Value"=w361) -> ()  [unwired: 2 in, 2 out]
                n233 = property on="buttonAcquisition" class="Bool (strict)"("DisabledEnum"=w358) -> ()  [unwired: 2 in, 2 out]
                n234 = local read "editTotalLowerLimit"() -> (w355:u8)
                n235 = property on="slideWaitLowerTime" class="Slide (strict)"("Scale.Maximum"=w355, "Scale.Minimum"=0.0 ("Scale.Range:Minimum"), "Scale.Increment"=1.0 ("Scale.Range:Increment"), "Value"=w355) -> ()  [unwired: 2 in, 2 out]
                n236 = local read "editTotalWaitLimit"() -> (w352:u8)
                n237 = property on="slideWaitTime" class="Slide (strict)"("Scale.Maximum"=w352, "Scale.Minimum"=0.0 ("Scale.Range:Minimum"), "Scale.Increment"=1.0 ("Scale.Range:Increment"), "Value"=w352) -> ()  [unwired: 2 in, 2 out]
                n238 = property on="buttonMotor" class="Bool (strict)"("DisabledEnum"=w358) -> ()  [unwired: 2 in, 2 out]
                n239 = property on="buttonBrake" class="Bool (strict)"("DisabledEnum"=w358) -> ()  [unwired: 2 in, 2 out]
                n240 = property on="editSetLowerLimit" class="DigNum (strict)"("DisabledEnum"=w358) -> ()  [unwired: 2 in, 2 out]
                n241 = property on="editSetUpperLimit" class="DigNum (strict)"("DisabledEnum"=w358) -> ()  [unwired: 2 in, 2 out]
              }
              frame #2 {
                n242 = local write "ledEnsaio"(TRUE ("ensaio")) -> ()
              }
            }
            n243 = disable-structure shown="Enabled" {
              frame Enabled {
                n244 = local write "ledInit2State"(TRUE ("ledReady")) -> ()
              }
              frame Disabled {
              }
            }
          }
          frame "motor acquire" {
            n245 = disable-structure shown="Enabled" {
              frame Enabled {
                n246 = local read "ledAcquireState"() -> (w374:bool)
                n247 = Not(x=w374) -> (.not. x?=w373:bool)
                n248 = local write "ledAcquireState"(w373) -> ()
              }
              frame Disabled {
              }
            }
            n249 = Wait (ms)(milliseconds to wait=u32 100) -> ()  [unwired: 1 out]
            n250 = disable-structure shown="Enabled" {
              disable-tunnel: [w371 w372] -> w364
              frame Enabled {
                n251 = property on="editSpeed" class="DigNum (strict)"() -> ("Value"=w371:dbl)  [unwired: 2 in, 2 out]
              }
              frame Disabled {
                n252 = property on="velocidade" class="DigNum (strict)"() -> ("Value"=w372:u32)  [unwired: 2 in, 2 out]
              }
            }
            n253 = property on="editSetUpperLimit" class="DigNum (strict)"() -> ("Value"=w363:u32)  [unwired: 2 in, 2 out]
            n254 = Greater Or Equal?(x=w364, y=w363) -> (x >= y?=w369:bool)
            n255 = case shown="True" w369 {
              selector: w369 -> [w375 _]
              tunnel: [w375 w376] -> w368
              frame False {
              }
              frame True {
                n256 = flat-sequence {
                  tunnel: [w381] -> w376
                  frame #0 {
                    n257 = local read "editCountUpperLimit"() -> (w379:u8)
                    n258 = Increment(x=w379) -> (x+1=w377:u8)
                    n259 = local write "editCountUpperLimit"(w377) -> ()
                    n260 = local read "editTotalUpperLimit"() -> (w378:u8)
                    n261 = Subtract(x=w378, y=w377) -> (x-y=w380:u8)
                    n262 = property on="sliderWaitUpperTime" class="Slide (strict)"("Value"=w380) -> ()  [unwired: 2 in, 2 out]
                  }
                  frame #1 {
                    n263 = local read "editCountUpperLimit"() -> (w383:u8)
                    n264 = local read "editTotalUpperLimit"() -> (w382:u8)
                    n265 = Greater Or Equal?(x=w383, y=w382) -> (x >= y?=w381:bool)
                  }
                }
              }
            }
            n266 = Select(t=testMachine."brake" ("testMachine"), s=w368, f=testMachine."motor acquire" ("testMachine")) -> (s? t:f=w365:T2)
          }
          frame "brake acquire" {
            n267 = disable-structure shown="Enabled" {
              frame Enabled {
                n268 = local read "ledAcquireState"() -> (w393:bool)
                n269 = Not(x=w393) -> (.not. x?=w392:bool)
                n270 = local write "ledAcquireState"(w392) -> ()
              }
              frame Disabled {
              }
            }
            n271 = Wait (ms)(milliseconds to wait=u32 100) -> ()  [unwired: 1 out]
            n272 = disable-structure shown="Enabled" {
              disable-tunnel: [w394 w395] -> w384
              frame Enabled {
                n273 = property on="editSpeed" class="DigNum (strict)"() -> ("Value"=w394:dbl)  [unwired: 2 in, 2 out]
              }
              frame Disabled {
                n274 = property on="velocidade" class="DigNum (strict)"() -> ("Value"=w395:u32)  [unwired: 2 in, 2 out]
              }
            }
            n275 = property on="editSetLowerLimit" class="DigNum (strict)"() -> ("Value"=w386:u32)  [unwired: 2 in, 2 out]
            n276 = Less Or Equal?(x=w384, y=w386) -> (x <= y?=w390:bool)
            n277 = case shown="True" w390 {
              selector: w390 -> [w396 _]
              tunnel: [w396 w397] -> w388
              frame False {
              }
              frame True {
                n278 = flat-sequence {
                  tunnel: [w403] -> w398
                  tunnel: w398 -> [w407]
                  tunnel: [w406] -> w397
                  frame #0 {
                    n279 = local read "editCountLowerLimit"() -> (w402:u8)
                    n280 = Increment(x=w402) -> (x+1=w401:u8)
                    n281 = local write "editCountLowerLimit"(w401) -> ()
                    n282 = local read "editTotalLowerLimit"() -> (w400:u8)
                    n283 = Subtract(x=w400, y=w401) -> (x-y=w399:u8)
                    n284 = property on="slideWaitLowerTime" class="Slide (strict)"("Value"=w399) -> ()  [unwired: 2 in, 2 out]
                  }
                  frame #1 {
                    n285 = local read "editCountLowerLimit"() -> (w405:u8)
                    n286 = local read "editTotalLowerLimit"() -> (w404:u8)
                    n287 = Greater Or Equal?(x=w405, y=w404) -> (x >= y?=w403:bool)
                  }
                  frame #2 {
                    n288 = case shown="True" w407 {
                      selector: w407 -> [w408 w409]
                      tunnel: [w408 w409] -> w406
                      frame False {
                      }
                      frame True {
                        # "- Desliga o freio"
                        n289 = local write "ledBrake"(FALSE ("freio")) -> ()
                      }
                    }
                  }
                }
              }
            }
            n290 = Select(t=testMachine."wait " ("testMachine"), s=w388, f=testMachine."brake acquire" ("testMachine")) -> (s? t:f=w385:T2)
          }
          frame "exit" {
          }
          frame "wait " {
            # "- Aguarda 0.5s \n- Atualiza o numero de ciclos"
            n291 = flat-sequence {
              tunnel: [w424] -> w412
              frame #0 {
                n292 = local read "editCountWaitLimit"() -> (w420:u8)
                n293 = Increment(x=w420) -> (x+1=w421:u8)
                n294 = local write "editCountWaitLimit"(w421) -> ()
                n295 = local read "editTotalWaitLimit"() -> (w423:u8)
                n296 = Subtract(x=w423, y=w421) -> (x-y=w422:u8)
                n297 = property on="slideWaitTime" class="Slide (strict)"("Value"=w422) -> ()  [unwired: 2 in, 2 out]
              }
              frame #1 {
                n298 = local read "editCountWaitLimit"() -> (w426:u8)
                n299 = local read "editTotalWaitLimit"() -> (w425:u8)
                n300 = Greater Or Equal?(x=w426, y=w425) -> (x >= y?=w424:bool)
              }
            }
            n301 = disable-structure shown="Enabled" {
              frame Enabled {
                n302 = local read "ledWaitState"() -> (w433:bool)
                n303 = Not(x=w433) -> (.not. x?=w432:bool)
                n304 = local write "ledBrakeState"(FALSE ("ledBrakeState")) -> ()
                n305 = local write "ledWaitState"(w432) -> ()
              }
              frame Disabled {
              }
            }
            n306 = Wait (ms)(milliseconds to wait=u32 100) -> ()  [unwired: 1 out]
            n307 = case shown="True" w412 {
              selector: w412 -> [w427 _]
              tunnel: [w427 w431] -> w413
              frame False {
              }
              frame True {
                n308 = local read "editSetNumberOfCycles"() -> (w429:u16)
                n309 = local read "editCurrCycleCtr"() -> (w428:u32)
                n310 = Greater Or Equal?(x=w428, y=w429) -> (x >= y?=w431:bool)
                n311 = Not(x=w431) -> (.not. x?=w430:bool)
                n312 = local write "ledEnsaio"(w430) -> ()
              }
            }
            n313 = Select(t=testMachine."motor" ("testMachine"), s=w412, f=testMachine."wait " ("testMachine")) -> (s? t:f=w414:T2)
            n314 = Select(t=testMachine."finish" ("testMachine"), s=w413, f=w414) -> (s? t:f=w418:T2)
          }
        }
        n315 = disable-structure shown="Enabled" {
          frame Disabled {
          }
          frame Enabled {
            n316 = local write "ledReadyState"(FALSE ("ledReady")) -> ()
            n317 = local write "ledRunningState"(TRUE ("ledReady")) -> ()
          }
        }
        n318 = local read "buttonStart"() -> (w296:bool)
        n319 = Select(t=mainMachine."running" ("mainMachine"), s=w296, f=mainMachine."blocked" ("mainMachine")) -> (s? t:f=w293:T1)
      }
      frame "blocked" {
        n320 = local read "buttonStart"() -> (w439:bool)
        n321 = Select(t=mainMachine."ready" ("mainMachine"), s=w439, f=mainMachine."blocked" ("mainMachine")) -> (s? t:f=w435:T1)
        n322 = local write "ledRunningState"(FALSE ("ledReady")) -> ()
        n323 = local write "ledBlockState"(TRUE ("ledReady")) -> ()
      }
      frame "finish" {
        n324 = local write "ledBlockState"(FALSE ("ledReady")) -> ()
      }
    }
    "mainMachine" <- w221
    "testMachine" <- w222
  }
  n325 = disable-structure shown="Disabled" {
    frame Disabled {
    }
    frame Enabled {
    }
  }
  "velocidade" <- "velocidade 2"
